vi "Move.vi"(8 "error in (no error)":errorcluster, 9 "Absolute (T)":bool=TRUE, 10 "Point":refnum<class "Point.lvclass">, 11 "Image in":refnum<class "Image.lvclass">) -> (0 "error out":errorcluster, 3 "Image out":refnum<class "Image.lvclass">)   [LabVIEW 2021, in "Picture2D.lvlib" / "Image.lvclass"]
uses:
  Image.lvclass
  Shape/Shape.lvclass
  Point/Point.lvclass
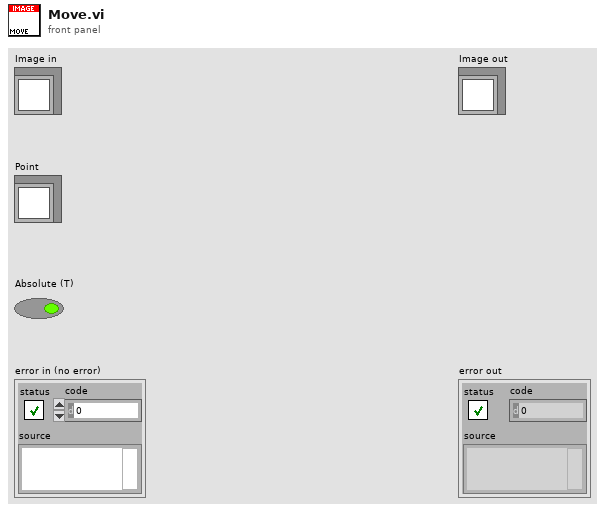
[diagram p1: front panel]
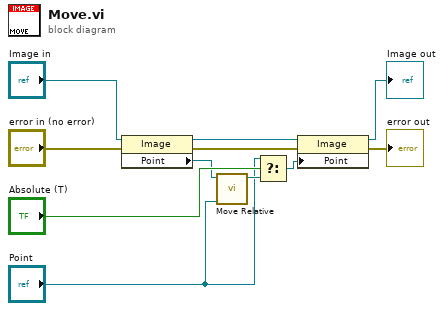
[diagram p0: block diagram]
diagram:
  n1 = property class="Image"(reference="Image in", error in="error in (no error)") -> (reference out=w4:refnum<class "Image.lvclass">, error out=w5:errorcluster, "Point"=w7:refnum<class "Point.lvclass">)
  n2 = call "Move Relative.vi"("Move"="Point", "Point"=w7) -> ("New Point"=w10:refnum<class "Point.lvclass">)  [unwired: 9 in]
  n3 = Select(t="Point", s="Absolute (T)", f=w10) -> (s? t:f=w1:refnum<class "Point.lvclass">)
  n4 = property class="Image"(reference=w4, error in=w5, "Point"=w1) -> (reference out=→"Image out":refnum<class "Image.lvclass">, error out=→"error out":errorcluster)
